vi "RT_Main.vi"() -> ()   [LabVIEW 2018]
uses:
  <vilib>/rvi/interface/nirviOpenFPGA/nirviOpenFPGA.xnode
  <vilib>/rvi/interface/nirviMethod/nirviMethod.xnode
  <vilib>/FPGAPlugInAG/Dynamic/niLvFpga_ReadFifo_Dynamic.vi
  <vilib>/rvi/errors/niLvFpgaMergeErrorWithErrorCode.vi
  <vilib>/rvi/interface/nirviReadWriteControl/nirviReadWriteControl.xnode
  <vilib>/rvi/interface/nirviCloseFPGA/nirviCloseFPGA.xnode
  <vilib>/FPGAPlugInAG/Dynamic/niLvFpga_Close_Dynamic.vi
  NiFpgaLv.dll
  <vilib>/Utility/error.llb/Error Cluster From Error Code.vi
  <vilib>/rvi/interface/Simulation/niFpgaSimulationCallBeginRW.vi
  <vilib>/rvi/errors/niLvFpgaAdjustHostInterfaceError.vi
  <vilib>/FPGAPlugInAG/Dynamic/niLvFpga_StartFifo_Dynamic.vi
  <vilib>/FPGAPlugInAG/Dynamic/niLvFpga_StopFifo_Dynamic.vi
  FPGA Bitfiles/DataLogging_FPGATarget_FPGADatalogMain_9gqMJBlA3fg.lvbitx
  FPGA_Datalog_Main.vi
  <vilib>/FPGAPlugInAG/myRIO-1900/niLvFpga_Open_myRIO-1900.vi
  <vilib>/rvi/interface/common/dynamic/niFpgaDynamicAddResources.vi
panel:
  out "FIFO Elements Remaining":u32=103
  in  "Acquisition Period (muS)":u32=1000 min=2
  out "appended path":path=path "c:/ni-rt/startup/10_10_19_11:40 AM_Trial.csv"
  out "Measurement 2":u16=34
  in  "Actuation 2":u16=250
  in  "Log data":bool=TRUE
  in  "Stop":bool=TRUE
  out "Measurement":u16[](graph)=[34, 34, 34, 34, 34, 34, 34, 34, 34, 34, 34, 34, 34, 34, 34, 34, 34, 34, 34, 34, 34, 34, 34, 34, 34, 34, 34, 34, 34, 34, 34, 34, 34, 34, 34, 34, 34, 34, 34, 34, 34, 34, 34, 34, 34, 34, 34, 34, 34, 34, 34, 34, 34, 34, 34, 34, 34, 34, 34, 34, 34, 34, 34, 34, 34, 34, 34, 34, 34, 34, 34, 34, 34, 34, 34, 34, 34, 34, 34, 34, 34, 34, 34, 34, 34, 34, 34, 34, 34, 34, 34, 34, 34, 34, 34, 34, 34, 34, 34, 34, 34, 34]
  out "Actuation":i16[](graph)=[250, 250, 250, 250, 250, 250, 250, 250, 250, 250, 250, 250, 250, 250, 250, 250, 250, 250, 250, 250, 250, 250, 250, 250, 250, 250, 250, 250, 250, 250, 250, 250, 250, 250, 250, 250, 250, 250, 250, 250, 250, 250, 250, 250, 250, 250, 250, 250, 250, 250, 250, 250, 250, 250, 250, 250, 250, 250, 250, 250, 250, 250, 250, 250, 250, 250, 250, 250, 250, 250, 250, 250, 250, 250, 250, 250, 250, 250, 250, 250, 250, 250, 250, 250, 250, 250, 250, 250, 250, 250, 250, 250, 250, 250, 250, 250, 250, 250, 250, 250, 250, 250]
  in  "File Name":string="Trial"
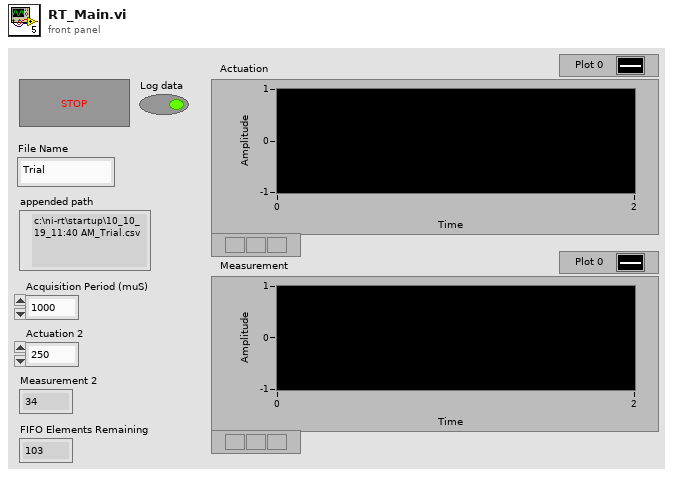
[diagram p1: front panel]
types:
  T1 = enum16{"open", "replace", "create", "open or create", "replace or create", "replace or create with confirmation"}
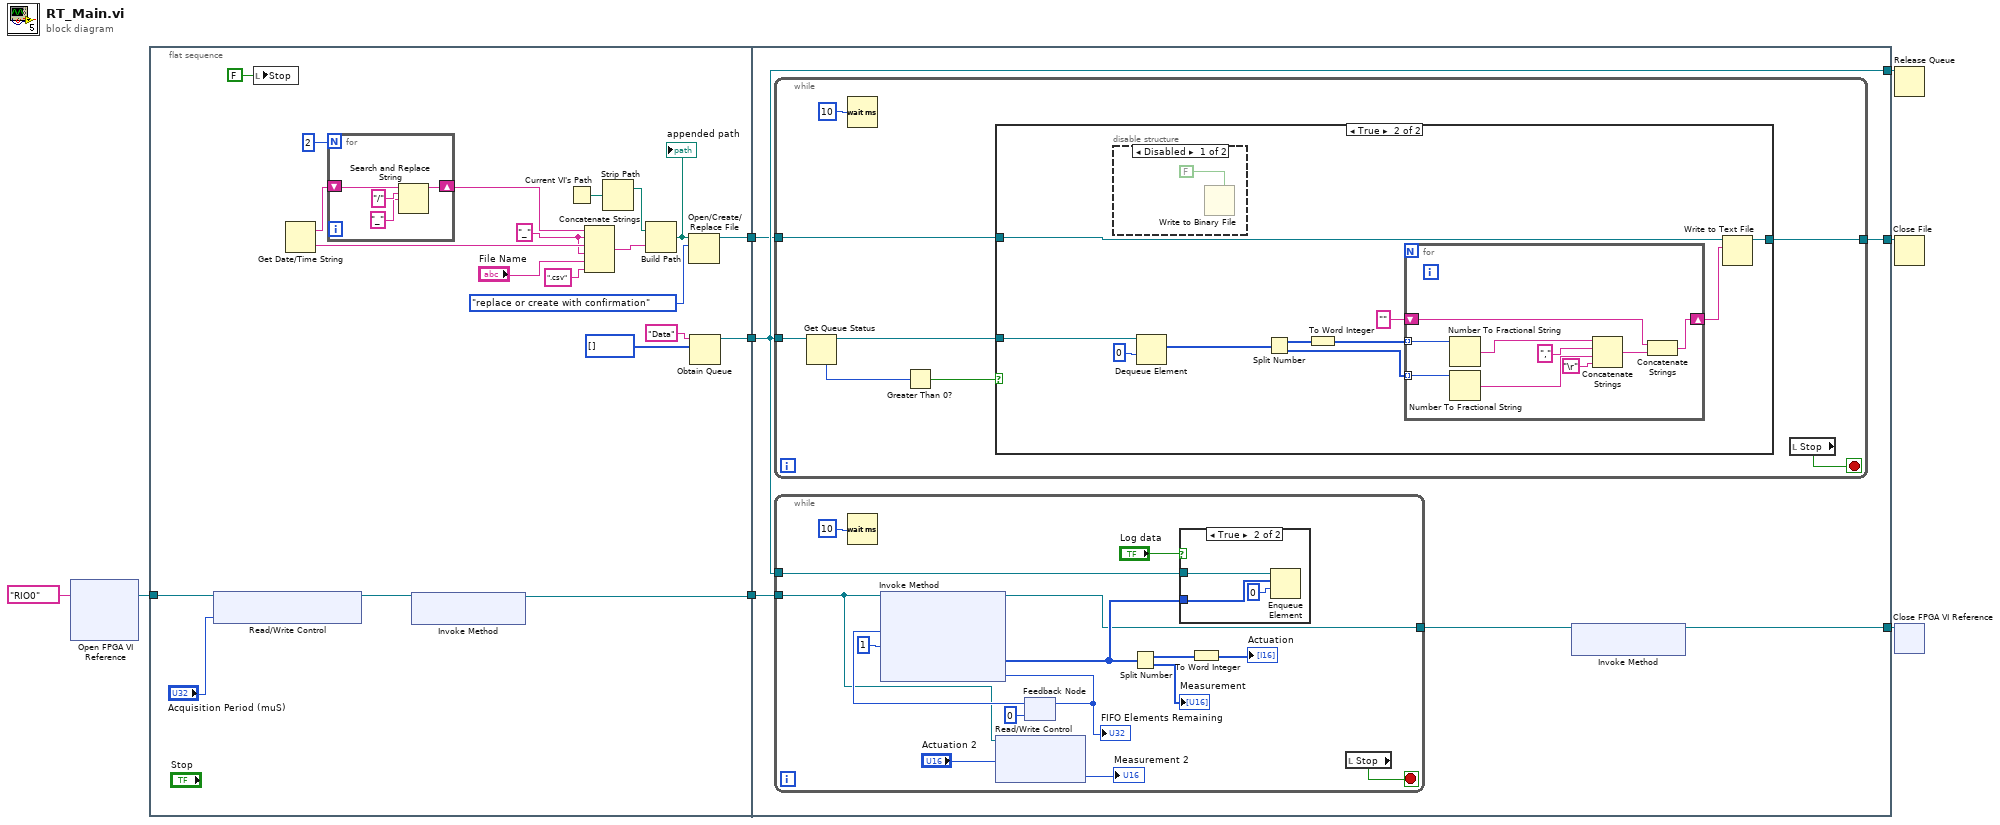
[diagram p0: block diagram]
diagram:
  n1 = xnode "Open FPGA VI Reference"("resource name"=tag "RIO0") -> ("FPGA VI Reference Out"=w7:refnum<k20>)  [unwired: 1 in, 1 out]
  n2 = flat-sequence {
    tunnel: w7 -> [w14]
    tunnel: [w12] -> w6
    tunnel: [w19] -> w5
    tunnel: [w16] -> w3
    tunnel: w6 -> [w39]
    tunnel: w5 -> [w38]
    tunnel: [w38] -> w4
    tunnel: w3 -> [w37]
    tunnel: [w34] -> w2
    tunnel: [w36] -> w1
    frame #0 {
      w11 = "_" ("replace string (\"\")")
      n3 = xnode "Read/Write Control"("FPGA VI Reference In"=w14, "Acquisition Period (muS)"="Acquisition Period (muS)") -> ("FPGA VI Reference Out"=w13:refnum<k20>)  [unwired: 1 in, 1 out]
      n4 = local write "Stop"(FALSE ("Stop")) -> ()
      n5 = Get Date/Time String() -> (date string=w27:string, time string=w24:string)  [unwired: 3 in]
      n6 = for {
        N: 2 -> [_]
        shift-right: [w31] -> w25
        shift-left: w27 -> [w30]
        n7 = Search and Replace String(input string=w30, search string="/", replace string="_" ("replace string (\"\")")) -> (result string=w31:string)  [unwired: 5 in, 3 out]
      }
      n8 = xnode "Invoke Method"("FPGA VI Reference In"=w13) -> ("FPGA VI Reference Out"=w12:refnum<k20>)  [unwired: 1 in, 1 out]
      n9 = Current VI's Path() -> (path=w29:path)
      n10 = Concatenate Strings(w25, w11, w24, w11, "File Name", ".csv" ("replace string (\"\")")) -> (w23:string)
      n11 = Strip Path(path=w29) -> (stripped path=w28:path)  [unwired: 1 out]
      n12 = Build Path(base path=w28, name or relative path=w23) -> (appended path=w17:path)
      "appended path" <- w17
      n13 = Open/Create/Replace File(file path (use dialog)=w17, operation (0:open)=T1."replace or create with confirmation") -> (refnum out=w16:refnum<file>)  [unwired: 4 in, 2 out]
      n14 = Obtain Queue(name (unnamed)="Data", element data type=u32[] [] ("Data")) -> (queue out=w19:refnum<queue>)  [unwired: 3 in, 2 out]
    }
    frame #1 {
      n15 = while {
        tunnel: w38 -> [w46]
        tunnel: [w42] -> w36
        tunnel: w37 -> [w41]
        stop <- w47 stop-if-true
        n16 = Get Queue Status(queue=w46) -> (queue out=w43:refnum<queue>, # elements in queue=w45:i32)  [unwired: 2 in, 6 out]
        n17 = Wait (ms)(milliseconds to wait=u32 10) -> ()  [unwired: 1 out]
        n18 = Greater Than 0?(x=w45) -> (x > 0?=w44:bool)
        n19 = case shown="True" w44 {
          tunnel: w43 -> [_ w57]
          tunnel: [w48 w53] -> w42
          tunnel: w41 -> [w48 w54]
          frame False {
          }
          frame True {
            n20 = disable-structure shown="Disabled" {
              frame Disabled {
                n21 = Write to Binary File(5:FALSE ("prepend array or string size? (T)")) -> ()  [unwired: 5 in, 3 out]
              }
              frame Enabled {
              }
            }
            n22 = Dequeue Element(queue=w57, timeout in ms (-1)=0) -> (element=w51:u32[])  [unwired: 1 in, 3 out]
            n23 = Split Number(x=w51) -> (hi(x)=w55:u16[], lo(x)=w52:u16[])
            n24 = To Word Integer(number=w55) -> (16bit integer=w50:i16[])
            n25 = for {
              shift-right: [w65] -> w49
              shift-left: "" -> [w64]
              tunnel: w52 -> [w61] mode=indexing
              tunnel: w50 -> [w60] mode=indexing
              n26 = Number To Fractional String(number=w60) -> (F-format string=w63:string)  [unwired: 3 in]
              n27 = Number To Fractional String(number=w61) -> (F-format string=w67:string)  [unwired: 3 in]
              n28 = Concatenate Strings(w63, "," ("string"), w67, "\r") -> (w66:string)
              n29 = Concatenate Strings(w64, w66) -> (w65:string)
            }
            n30 = Write to Text File(file (use dialog)=w54, text=w49) -> (refnum out=w53:refnum<file>)  [unwired: 2 in, 2 out]
          }
        }
        n31 = local read "Stop"() -> (w47:bool)
      }
      n32 = while {
        tunnel: w39 -> [w73]
        tunnel: w38 -> [w81]
        tunnel: [w74] -> w35
        stop <- w76 stop-if-true
        n33 = Wait (ms)(milliseconds to wait=u32 10) -> ()  [unwired: 1 out]
        n34 = xnode "Read/Write Control"("FPGA VI Reference In"=w73, "Actuation"="Actuation 2") -> ("Measurement"=→"Measurement 2":u16)  [unwired: 1 in, 2 out]
        n35 = feedback #1(u32 0 ("Elements Remaining")) -> (w83:u32)
        n36 = xnode "Invoke Method"("FPGA VI Reference In"=w73, "Number of Elements"=w83, "Timeout (ms)"=1) -> ("FPGA VI Reference Out"=w74:refnum<k20>, "Data"=w80:u32[], "Elements Remaining"=w84:u32)  [unwired: 1 in, 1 out]
        "FIFO Elements Remaining" <- w84
        n37 = feedback-in #1(w84) -> ()
        n38 = Split Number(x=w80) -> (hi(x)=w77:u16[], lo(x)=→"Measurement":u16[])
        n39 = case shown="True" "Log data" {
          tunnel: w81 -> [_ w86]
          tunnel: w80 -> [_ w85]
          frame False {
          }
          frame True {
            n40 = Enqueue Element(queue=w86, element=w85, timeout in ms (-1)=0) -> ()  [unwired: 1 in, 3 out]
          }
        }
        n41 = To Word Integer(number=w77) -> (16bit integer=→"Actuation":i16[])
        n42 = local read "Stop"() -> (w76:bool)
      }
      n43 = xnode "Invoke Method"("FPGA VI Reference In"=w35) -> ("FPGA VI Reference Out"=w34:refnum<k20>)  [unwired: 1 in, 1 out]
    }
  }
  n44 = Release Queue(queue=w4) -> ()  [unwired: 2 in, 3 out]
  n45 = Close File(refnum=w1) -> ()  [unwired: 1 in, 2 out]
  n46 = xnode "Close FPGA VI Reference"("FPGA VI Reference In"=w2) -> ()  [unwired: 1 in, 1 out]
